vi "Get Module Running State.vi"() -> (3 "Module Running State":T1)   [LabVIEW 2020, in "MQTT_Client.lvlib"]
doc: "Determine if the cloneable module is not running, running as cloneable, or running as singleton.\n_____\nBased on Delacor QMH Project Template 5.0.0.82."
uses:
  MQTT_Client.lvlib
  Module Running State--enum.ctl
  Clone Registration/Clone Registration.lvlib
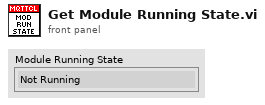
[diagram p1: front panel]
types:
  T1 = typedef "MQTT_Client.lvlib/Module Running State--enum.ctl" = enum16{"Not Running", "Running as Cloneable", "Running as Singleton"}
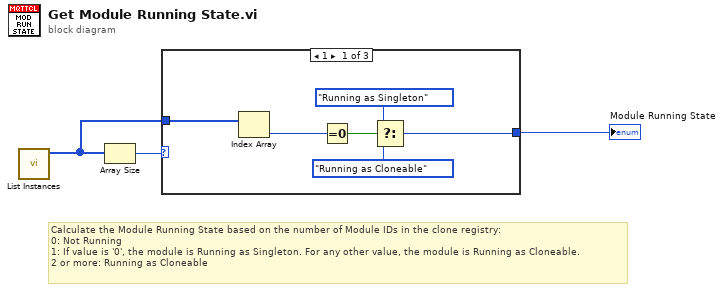
[diagram p0: block diagram]
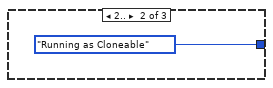
[diagram p2: hidden frame]
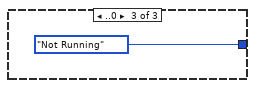
[diagram p3: hidden frame]
diagram:
  # "Calculate the Module Running State based on the number of Module IDs in the clone registry:\n0: Not Running\n1: If value is '0', the module is Running as Singleton. For any other value, the module is Running as Cloneable.\n2 or more: Running as Cloneable"
  n1 = call "List Instances.vi"() -> ("Module IDs"=w1:i32[])  [unwired: 7 in, 4 out]
  n2 = Array Size(array=w1) -> (size(s)=w3:i32)
  n3 = case shown="1" w3 {
    tunnel: [w4 Module_Running_State--enum."Running as Cloneable" ("Module Running State") Module_Running_State--enum."Not Running" ("Module Running State")] -> w2
    tunnel: w1 -> [w9 _ _]
    frame 1 {
      n4 = Index Array(array=w9) -> (element=w8:i32)  [unwired: 1 in]
      n5 = Equal To 0?(x=w8) -> (x = 0?=w7:bool)
      n6 = Select(t=Module_Running_State--enum."Running as Singleton" ("Module Running State"), s=w7, f=Module_Running_State--enum."Running as Cloneable" ("Module Running State")) -> (s? t:f=w4:T1)
    }
    frame 2.. {
    }
    frame ..0 {
    }
  }
  "Module Running State" <- w2
